vi "picoquant_read_buffer.vi"(8 "error in (no error)":errorcluster, 11 "picoharp in":refnum<class "picoharp.lvclass">) -> (0 "error out":errorcluster, 2 "new_data":u32[](array[numeric]), 3 "picoharp out":refnum<class "picoharp.lvclass">)   [LabVIEW 2015, in "picoharp.lvclass"]
uses:
  picoharp.lvclass
  picoharp.lvclass/picoharp.ctl
  phlib.dll
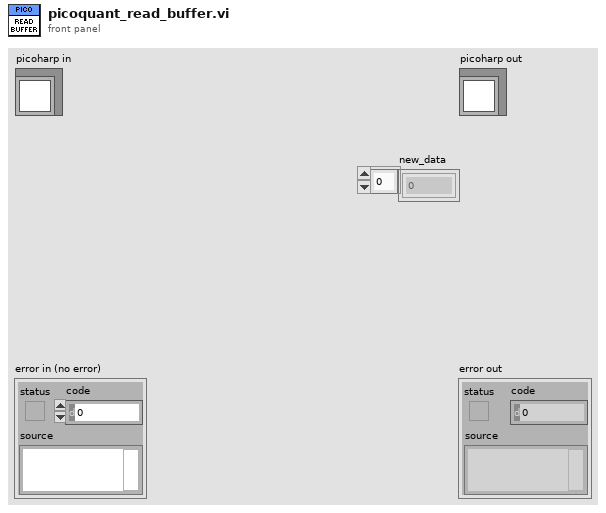
[diagram p1: front panel]
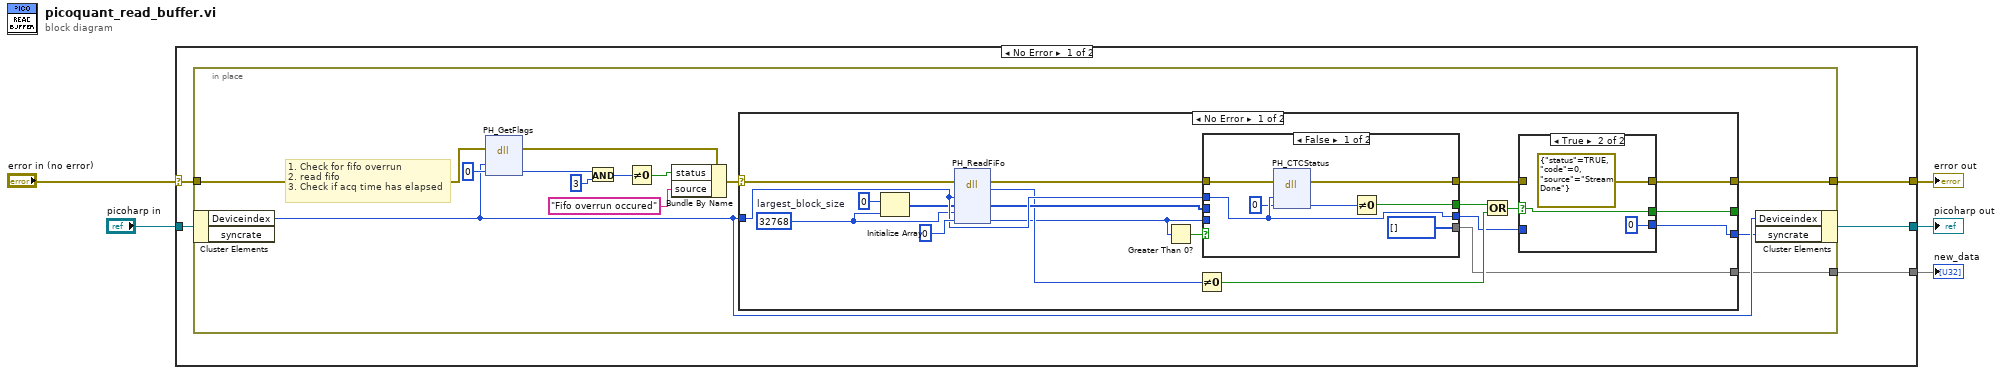
[diagram p0: block diagram]
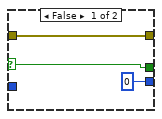
[diagram p2: hidden frame]
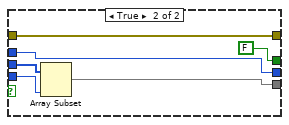
[diagram p3: hidden frame]
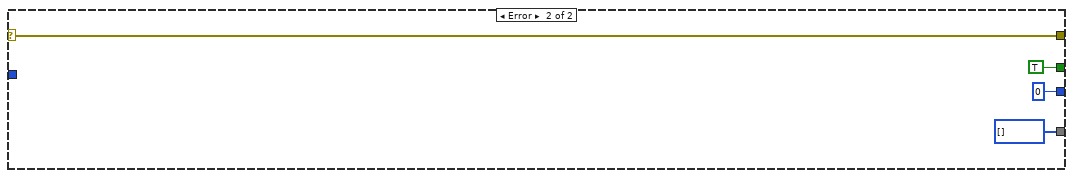
[diagram p4: hidden frame]
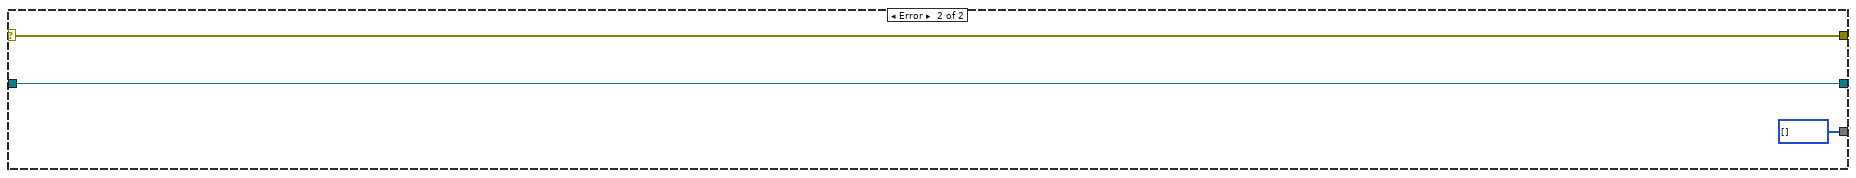
[diagram p5: hidden frame]
diagram:
  n1 = case shown="No Error" "error in (no error)" {
    selector: "error in (no error)" -> [w9 w69]
    tunnel: [w8 w69] -> w3
    tunnel: [w7 w68] -> w2
    tunnel: "picoharp in" -> [w10 w68]
    tunnel: [w6 u32[] []] -> w1
    frame No Error {
      n2 = in-place {
        in-place-border: w9 -> [w23]
        in-place-border: [w11] -> w8
        in-place-border: [w14] -> w6
        # "1. Check for fifo overrun\n2. read fifo\n3. Check if acq time has elapsed"
        n3 = in-place-cluster #1(w10) -> ("Deviceindex"=w19:i32)  [unwired: 1 out]
        n4 = dll-call lib="phlib.dll" fn="PH_GetFlags" label="pH_GetFlags"(error in=w23, "devidx"=w19, "flags"=0) -> (error out=w18:errorcluster, "flags"=w21:i32)  [unwired: 4 in, 1 out]
        n5 = And(x=w21, y=3) -> (x .and. y?=w16:i32)
        n6 = Not Equal To 0?(x=w16) -> (x != 0?=w12:bool)
        n7 = Bundle By Name(cluster=w18, "status"=w12, "source"="Fifo overrun occured") -> (w17:errorcluster)
        n8 = case shown="No Error" w17 {
          selector: w17 -> [w34 w65]
          tunnel: w19 -> [w40 _]
          tunnel: [w36 w65] -> w11
          tunnel: [w35 TRUE] -> _
          tunnel: [w25 0 ("syncrate")] -> w15
          tunnel: [w24 u32[] []] -> w14
          frame No Error {
            w28 = 32768  # largest_block_size
            n9 = Initialize Array(u32 0 ("element"), w28) -> (w27:u32[])
            n10 = dll-call lib="phlib.dll" fn="PH_ReadFiFo" label="pH_ReadFiFo"(error in=w34, "devidx"=w40, "buffer"=w27, "blocksize"=w28, "nactual"=0) -> (error out=w41:errorcluster, "return type"=w33:i32, "buffer"=w38:u32[], "nactual"=w30:i32)  [unwired: 4 in, 1 out]
            n11 = Greater Than 0?(x=w30) -> (x > 0?=w42:bool)
            n12 = Not Equal To 0?(x=w33) -> (x != 0?=w32:bool)
            n13 = case shown="False" w42 {
              tunnel: w41 -> [w56 w58]
              tunnel: [w55 w58] -> w31
              tunnel: w40 -> [w54 w59]
              tunnel: [w51 FALSE] -> w39
              tunnel: w38 -> [_ w61]
              tunnel: w30 -> [_ w60]
              tunnel: [w54 w59] -> w26
              tunnel: [u32[] [] w57] -> w24
              frame False {
                n14 = dll-call lib="phlib.dll" fn="PH_CTCStatus" label="pH_CTCStatus"(error in=w56, "devidx"=w54, "status"=0) -> (error out=w55:errorcluster, "status"=w52:i32)  [unwired: 4 in, 1 out]
                n15 = Not Equal To 0?(x=w52) -> (x != 0?=w51:bool)
              }
              frame True {
                n16 = Array Subset(array=w61, length=w60) -> (w57:u32[])  [unwired: 1 in]
              }
            }
            n17 = Or(x=w39, y=w32) -> (x .or. y?=w37:bool)
            n18 = case shown="True" w37 {
              selector: w37 -> [w45 w49]
              tunnel: w31 -> [w46 _]
              tunnel: [w46 errorcluster {"status"=TRUE, "code"=0, "source"="Stream Done"} ("error out")] -> w36
              tunnel: [w45 w49] -> w35
              tunnel: w26 -> [_ _]
              tunnel: [0 ("syncrate") 0 ("syncrate")] -> w25
              frame False {
              }
              frame True {
              }
            }
          }
          frame Error {
          }
        }
        n19 = in-place-cluster #1("Deviceindex"=w19, "syncrate"=w15) -> (w7:refnum<class "picoharp.lvclass">)
      }
    }
    frame Error {
    }
  }
  "error out" <- w3
  "picoharp out" <- w2
  "new_data" <- w1
